vi "myrio_find_usb.vi"() -> (0 "Found?":bool, 2 "Free Capacity [MB]":u32, 3 "Largest USB Partition Path":path)   [LabVIEW 2019]
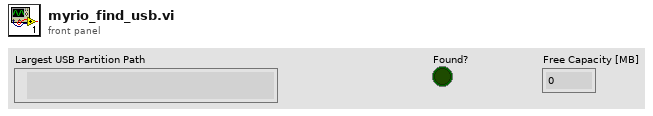
[diagram p1: front panel]
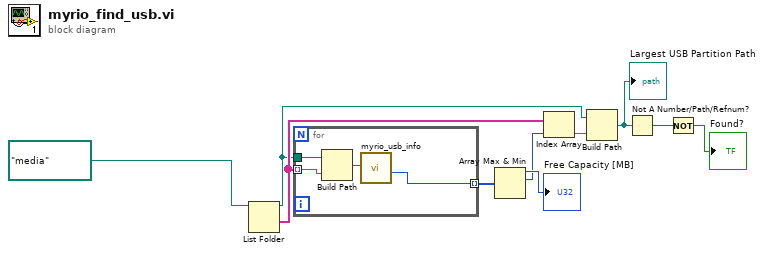
[diagram p0: block diagram]
diagram:
  n1 = List Folder(path=path "/media") -> (path out=w5:path, folder names=w7:string[])  [unwired: 3 in, 2 out]
  n2 = for {
    tunnel: w5 -> [w14]
    tunnel: w7 -> [w13] mode=indexing
    tunnel: [w11] -> w9 mode=indexing
    n3 = Build Path(base path=w14, name or relative path=w13) -> (appended path=w12:path)
    n4 = call "myrio_usb_info.vi"("Path"=w12) -> ("Free Capacity [MB]"=w11:u32)  [unwired: 5 in, 5 out]
  }
  n5 = Array Max & Min(array=w9) -> (max value=→"Free Capacity [MB]":u32, max index (indices)=w6:i32)  [unwired: 2 out]
  n6 = Index Array(array=w7, index=w6) -> (element=w4:string)
  n7 = Build Path(base path=w5, name or relative path=w4) -> (appended path=w3:path)
  "Largest USB Partition Path" <- w3
  n8 = Not A Number/Path/Refnum?(number/path/refnum=w3) -> (NaN/Path/Refnum?=w2:bool)
  n9 = Not(x=w2) -> (.not. x?=→"Found?":bool)
